vi "DAQ_SynchronousStart.vi"(0 "reference in":refnum<class "NI_DAQ.lvclass">, 5 "error in (no error)":errorcluster) -> (14 "reference out":refnum<class "NI_DAQ.lvclass">, 19 "error out":errorcluster)   [LabVIEW 2020, in "DAQ.lvlib" / "NI_DAQ.lvclass"]
uses:
  NI_DAQ.lvclass
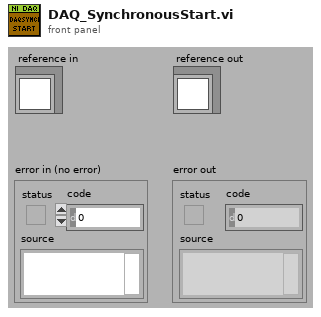
[diagram p1: front panel]
types:
  T1 = typedef "DAQ.lvlib/NI_DAQ.lvclass/ObjectAttributesRef.ctl" = refnum<data-value>
  T2 = typedef "DAQ.lvlib/NI_DAQ.lvclass/ObjectAttributes.ctl" = cluster{"MyAttribute":dbl, "DAQ_AI_task_out":refnum<k21>, "counter_task_out":refnum<k21>[]}
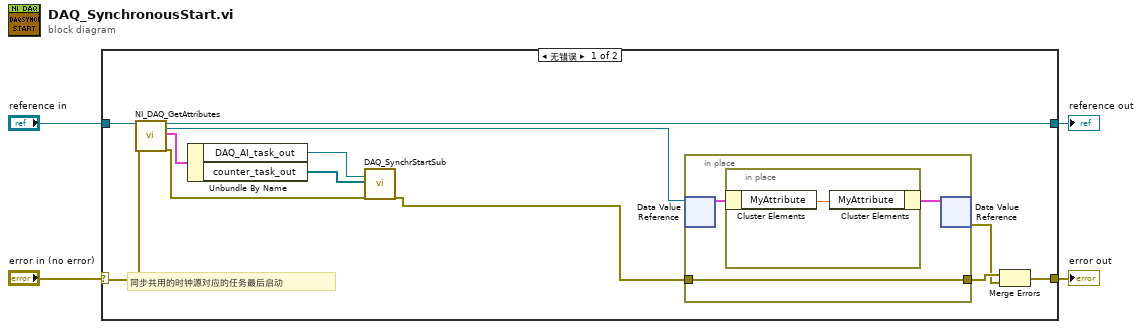
[diagram p0: block diagram]
diagram:
  n1 = case shown="无错误" "error in (no error)" {
    selector: "error in (no error)" -> [w13 w22]
    tunnel: [w16 w22] -> w3
    tunnel: [w14 w21] -> w1
    tunnel: "reference in" -> [w15 w21]
    frame No Error {
      # "同步共用的时钟源对应的任务最后启动"
      n2 = call "NI_DAQ_GetAttributes.vi"("reference in"=w15, "error in (no error)"=w13) -> ("reference out"=w14:refnum<class "NI_DAQ.lvclass">, "attributes ref"=w9:T1, "attributes"=w12:T2, "error out"=w6:errorcluster)  [unwired: 14 in]
      n3 = Unbundle By Name(w12) -> ("DAQ_AI_task_out"=w8:refnum<k21>, "counter_task_out"=w7:refnum<k21>[])
      n4 = call "DAQ_SynchrStartSub.vi"("DAQ_AI_task_out"=w8, "counter_task_out"=w7, "error in"=w6) -> ("error out"=w5:errorcluster)  [unwired: 16 in]
      n5 = in-place {
        in-place-border: w5 -> [w17]
        in-place-border: [w17] -> w11
        n6 = in-place-dvr #1(w9) -> (w18:T2)  [unwired: 1 out]
        n7 = in-place {
          n8 = in-place-cluster #2(w18) -> ("MyAttribute"=w20:dbl)
          n9 = in-place-cluster #2("MyAttribute"=w20) -> (w19:T2)
        }
        n10 = in-place-dvr #1(w19) -> (w10:errorcluster)  [unwired: 1 out]
      }
      n11 = Merge Errors(w11, w10) -> (w16:errorcluster)
    }
    frame Error {
    }
  }
  "error out" <- w3
  "reference out" <- w1
